vi "LS372_set_main_measuring_channel.vi"(0 "VISA resource name":refnum<visa-resource-name>, 1 "Channel":dbl) -> (3 "dup VISA":refnum<visa-resource-name>)   [LabVIEW 2019]
uses:
  Instrument_Setup.vi
  Equipment/Lake Shore 372/Lake Shore 372.lvlib
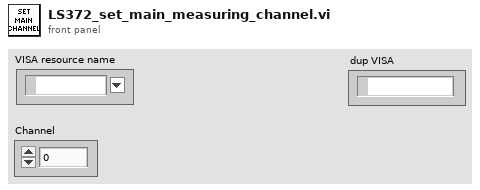
[diagram p1: front panel]
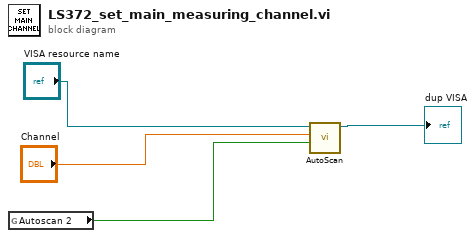
[diagram p0: block diagram]
diagram:
  n1 = global read "Instrument_Setup.vi" "Autoscan 2"() -> (w1:bool)
  n2 = call "AutoScan.vi"("Autoscan (F: Off)"=w1, "Channel (1:1)"="Channel", "VISA resource name"="VISA resource name") -> ("VISA resource name out"=→"dup VISA":refnum<visa-resource-name>)  [unwired: 7 in, 1 out]
